vi "Frame Get Title.vi"(8 "error in (no error)":errorcluster, 11 "IDE simple in":refnum<class "Main Panel.lvclass">) -> (0 "error out":errorcluster, 2 "Frame Title":T1, 3 "IDE simple out":refnum<class "Main Panel.lvclass">)   [LabVIEW 2018, in "Main Panel.lvlib" / "Main Panel.lvclass"]
uses:
  Main Panel.lvclass
  Frame Analizer/frame title.ctl
  Main Panel.lvclass/Main Panel.ctl
  Frame Analizer/Data Parser.lvclass
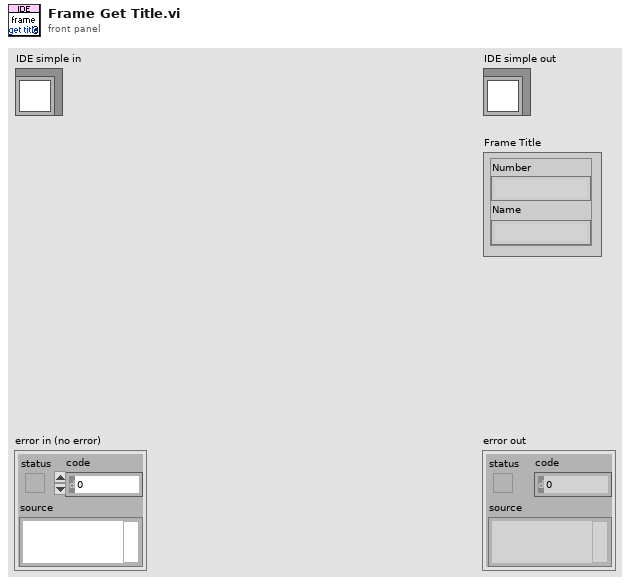
[diagram p1: front panel]
types:
  T1 = typedef "Data Parser.lvclass/frame title.ctl" = cluster{"Number":string, "Name":string}
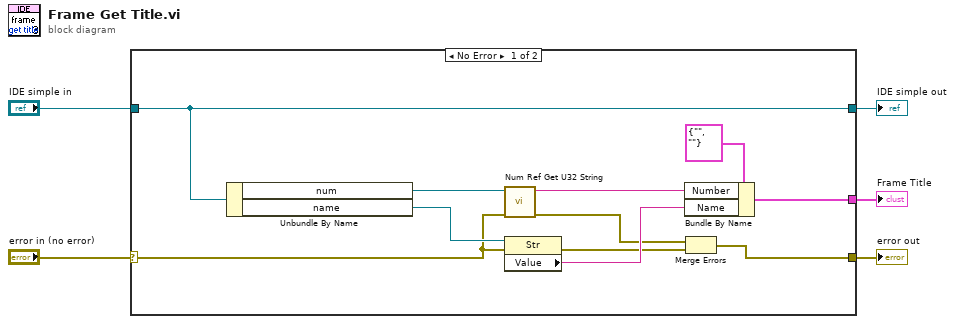
[diagram p0: block diagram]
diagram:
  n1 = case shown="No Error" "error in (no error)" {
    selector: "error in (no error)" -> [w6 w18]
    tunnel: [w15 w18] -> w4
    tunnel: [w16 w17] -> w2
    tunnel: "IDE simple in" -> [w16 w17]
    tunnel: [w14 _] -> w1
    frame No Error {
      n2 = Unbundle By Name(w16) -> ("num"=w12:refnum<vi>, "name"=w10:refnum<vi>)
      n3 = call "Num Ref Get U32 String.vi"("error in (no error)"=w6, "U32 Ref"=w12) -> ("error out"=w8:errorcluster, "Value string"=w11:string)  [unwired: 8 in]
      n4 = property class="Str"(reference=w10, error in=w6) -> (error out=w7:errorcluster, "Value"=w9:string)  [unwired: 1 out]
      n5 = Bundle By Name(cluster=T1 {"Number"="", "Name"=""} ("frame title 2"), "Number"=w11, "Name"=w9) -> (w14:T1)
      n6 = Merge Errors(w8, w7) -> (w15:errorcluster)
    }
    frame Error {
    }
  }
  "error out" <- w4
  "IDE simple out" <- w2
  "Frame Title" <- w1
